vi "Get State from Routing Channel.vi"(8 "error in":errorcluster, 10 "state":string, 11 "routing channel in":T3 format="%.0x") -> (0 "error out":errorcluster, 2 "state and connections":T1, 3 "routing channel out":T3=18446744073709551615 format="%.0x")   [LabVIEW 2020, in "Routing and Faulting Scripting.lvlib"]
doc: "Gets the configuration of the routing channel state with the specified name."
uses:
  Routing and Faulting Scripting.lvlib
  <vilib>/NI VeriStand/Custom Device API/Custom Device Item Ref.ctl
  Shared/Routing State.ctl
  Shared/Connection.ctl
  NationalInstruments.VeriStand.SystemDefinitionAPI
  Constants/Scripting Constants.vi
  Dependencies.llb/Routing and Faulting Shared.lvlib
  <vilib>/NI VeriStand/Custom Device API/Custom Device API.lvlib
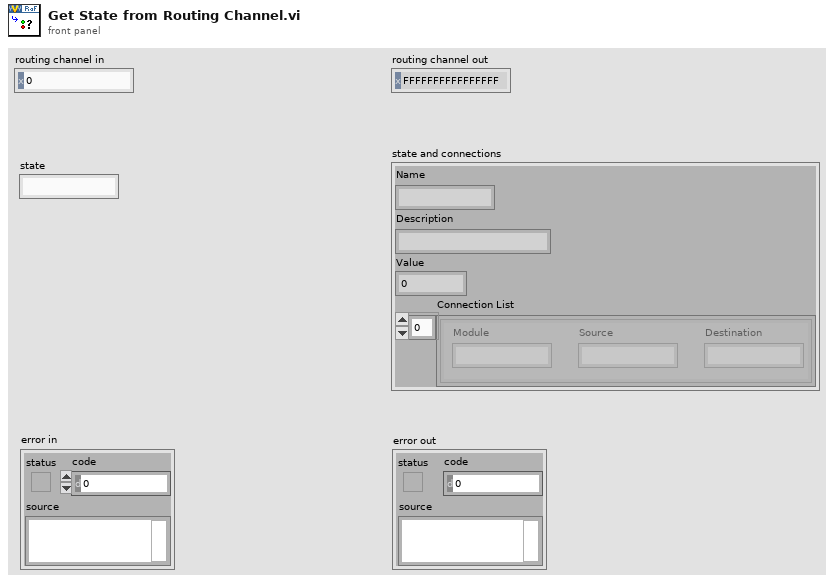
[diagram p1: front panel]
types:
  T1 = typedef "Routing and Faulting Shared.lvlib/Routing State.ctl" = cluster{"Name":string, "Description":string, "Value":i32, "Connection List":T2[]}
  T2 = typedef "Routing and Faulting Shared.lvlib/Connection.ctl" = cluster{"Module":string, "Source":string, "Destination":string}
  T3 = typedef "Custom Device API.lvlib/Custom Device Item Ref.ctl" = u64
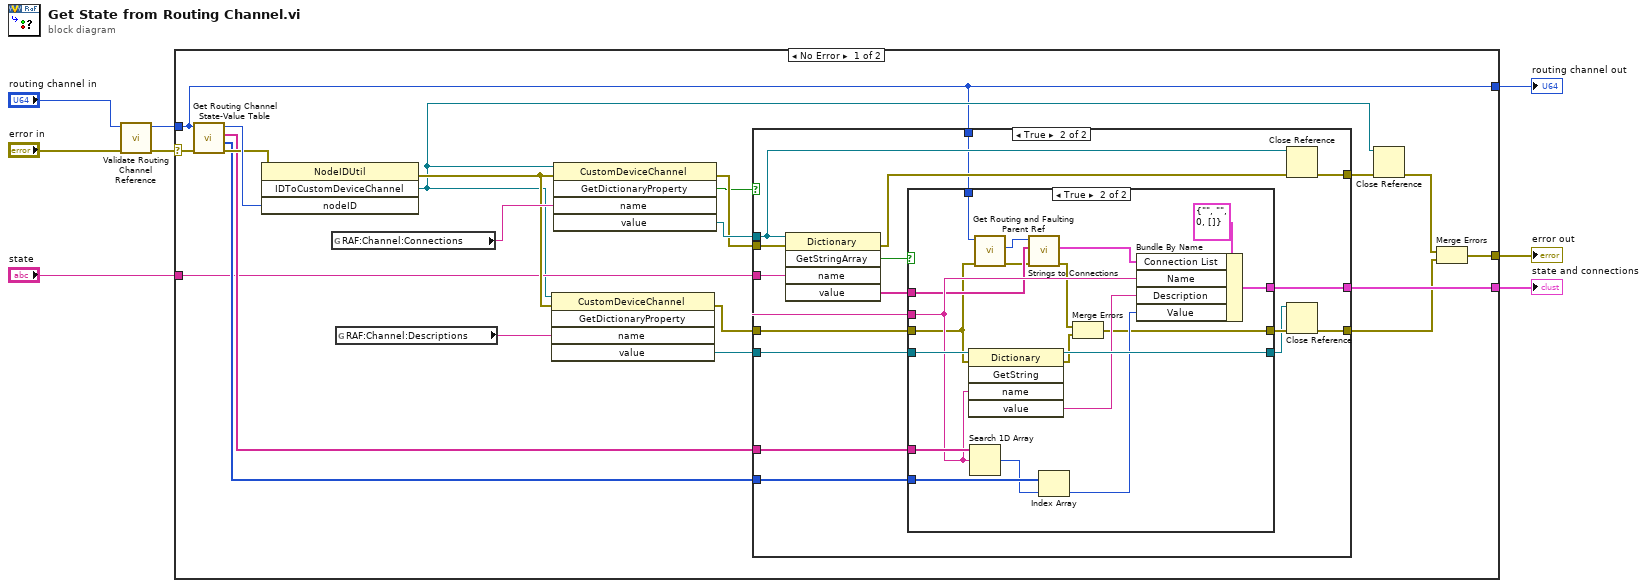
[diagram p0: block diagram]
diagram:
  n1 = call "Validate Routing Channel Reference.vi"("error in"="error in", "routing channel in"="routing channel in") -> ("error out"=w3:errorcluster, "routing channel out"=w1:T3)  [unwired: 8 in]
  n2 = case shown="No Error" w3 {
    selector: w3 -> [w27 w70]
    tunnel: [w15 w70] -> w5
    tunnel: w1 -> [w9 w69]
    tunnel: [w9 w69] -> w4
    tunnel: [w29 _] -> w6
    tunnel: "state" -> [w12 _]
    frame No Error {
      n3 = call "Get Routing Channel State-Value Table.vi"("error in"=w27, "routing channel in"=w9) -> ("error out"=w26:errorcluster, "state values"=w24:i32[], "state names"=w25:string[], "routing channel out"=w28:T3)  [unwired: 6 in]
      n4 = invoke class="NodeIDUtil" method="IDToCustomDeviceChannel"(error in=w26, "nodeID"=w28) -> (error out=w20:errorcluster, "IDToCustomDeviceChannel"=w11:refnum<k24>)  [unwired: 2 in, 2 out]
      n5 = global read "Scripting Constants.vi" "RAF:Channel:Connections"() -> (w23:string)
      n6 = global read "Scripting Constants.vi" "RAF:Channel:Descriptions"() -> (w22:string)
      n7 = invoke class="CustomDeviceChannel" method="GetDictionaryProperty"(reference=w11, error in=w20, "name"=w22) -> (error out=w19:errorcluster, "value"=w21:refnum<k24>)  [unwired: 2 in, 3 out]
      n8 = invoke class="CustomDeviceChannel" method="GetDictionaryProperty"(reference=w11, error in=w20, "name"=w23) -> (error out=w13:errorcluster, "GetDictionaryProperty"=w10:bool, "value"=w14:refnum<k24>)  [unwired: 2 in, 2 out]
      n9 = case shown="True" w10 {
        tunnel: [_ w47] -> w29
        tunnel: w25 -> [_ w46]
        tunnel: w24 -> [_ w45]
        tunnel: w21 -> [_ w44]
        tunnel: w19 -> [w30 w43]
        tunnel: [w31 w41] -> w18
        tunnel: [w30 w40] -> w16
        tunnel: w14 -> [_ w33]
        tunnel: w13 -> [w31 w39]
        tunnel: w12 -> [_ w36]
        tunnel: w9 -> [_ w32]
        frame False {
        }
        frame True {
          n10 = invoke class="Dictionary" method="GetStringArray"(reference=w33, error in=w39, "name"=w36) -> (error out=w37:errorcluster, "GetStringArray"=w35:bool, "value"=w38:string[])  [unwired: 2 in, 2 out]
          n11 = case shown="True" w35 {
            tunnel: [_ w68] -> w47
            tunnel: w46 -> [_ w67]
            tunnel: w45 -> [_ w66]
            tunnel: w44 -> [w49 w65]
            tunnel: [w49 w64] -> w34
            tunnel: w43 -> [w48 w53]
            tunnel: [w48 w52] -> w42
            tunnel: w38 -> [_ w58]
            tunnel: w36 -> [_ w59]
            tunnel: w32 -> [_ w56]
            frame False {
            }
            frame True {
              n12 = invoke class="Dictionary" method="GetString"(reference=w65, error in=w53, "name"=w59) -> (reference out=w64:refnum<k24>, error out=w50:errorcluster, "value"=w60:string)  [unwired: 2 in, 2 out]
              n13 = Search 1D Array(1D array=w67, element=w59) -> (index of element=w62:i32)  [unwired: 1 in]
              n14 = call "Get Routing and Faulting Parent Ref.vi"("error in"=w53, "routing and faulting child in"=w56) -> ("error out"=w54:errorcluster, "routing and faulting"=w55:T3)  [unwired: 7 in, 1 out]
              n15 = call "Strings to Connections.vi"("error in"=w54, "connection strings"=w58, "routing and faulting in"=w55) -> ("error out"=w51:errorcluster, "connection list"=w57:T2[])  [unwired: 6 in, 1 out]
              n16 = Index Array(array=w66, index=w62) -> (element=w61:i32)
              n17 = Merge Errors(w51, w50) -> (w52:errorcluster)
              n18 = Bundle By Name(cluster=T1 {"Name"="", "Description"="", "Value"=0, "Connection List"=[]} ("Routing State"), "Connection List"=w57, "Name"=w59, "Description"=w60, "Value"=w61) -> (w68:T1)
            }
          }
          n19 = Close Reference(reference=w33, error in (no error)=w37) -> (error out=w41:errorcluster)
          n20 = Close Reference(reference=w34, error in (no error)=w42) -> (error out=w40:errorcluster)
        }
      }
      n21 = Close Reference(reference=w11, error in (no error)=w18) -> (error out=w17:errorcluster)
      n22 = Merge Errors(w17, w16) -> (w15:errorcluster)
    }
    frame Error {
    }
  }
  "routing channel out" <- w4
  "error out" <- w5
  "state and connections" <- w6
